vi "Set Dialog Title.vi"(8 "error in":errorcluster, 10 "Dialog Title":string, 11 "Plain Parent in":refnum<class "Plain Parent.lvclass">) -> (0 "error out":errorcluster, 3 "Plain Parent out":refnum<class "Plain Parent.lvclass">)   [LabVIEW 2021, in "Pop-Up.lvlib" / "Plain Parent.lvclass"]
doc: "data member access VI: write the dialog title text for the plain pop up"
uses:
  Plain Parent.lvclass
  Plain Parent.lvclass/Plain Parent.ctl
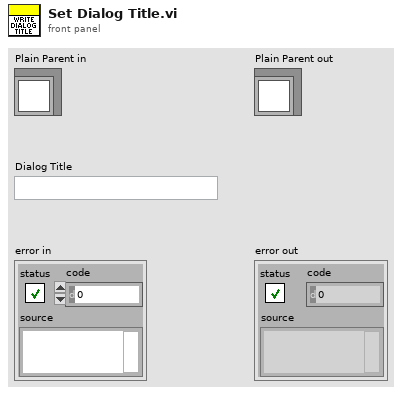
[diagram p1: front panel]
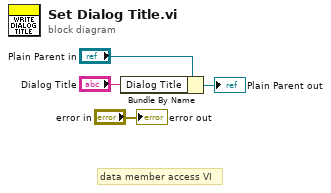
[diagram p0: block diagram]
diagram:
  # "data member access VI"
  n1 = Bundle By Name(cluster="Plain Parent in", "Dialog Title"="Dialog Title") -> (→"Plain Parent out":refnum<class "Plain Parent.lvclass">)
  "error out" <- "error in"
